vi "Pause Screen.vi"(8 "error in (no error)":errorcluster, 10 "Pause screen?":bool, 11 "VISA resource name":refnum<visa-resource-name>) -> (0 "error out":errorcluster, 3 "VISA resource name out":refnum<visa-resource-name>)   [LabVIEW 2017, in "Sefram DAS220.lvlib"]
doc: "Freeze/unfreeze the screen in graphic F(t) mode."
uses:
  <instrlib>/Sefram DAS220/Sefram DAS220.lvlib
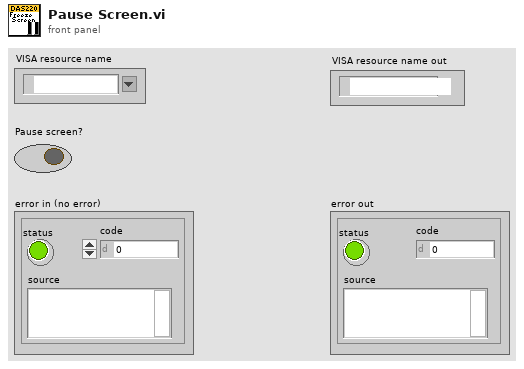
[diagram p1: front panel]
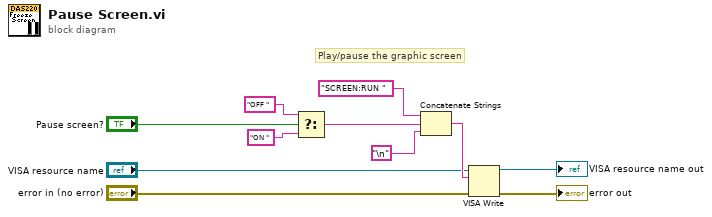
[diagram p0: block diagram]
diagram:
  # "Play/pause the graphic screen"
  n1 = Select(t="OFF " ("string"), s="Pause screen?", f="ON " ("string")) -> (s? t:f=w3:string)
  n2 = Concatenate Strings("SCREEN:RUN " ("string"), w3, "\n") -> (w11:string)
  n3 = VISA Write(VISA resource name="VISA resource name", write buffer=w11, error in (no error)="error in (no error)") -> (VISA resource name out=→"VISA resource name out":refnum<visa-resource-name>, error out=→"error out":errorcluster)  [unwired: 1 out]
